vi "MB Registers Manager Write.vi"(5 "Data Reference":T2, 6 "Bits In":bool[](array[boolean]), 8 "error in (no error)":errorcluster, 9 "Words In":u16[](array[numeric]), 10 "Table":T1(ring), 11 "Start Address":u16) -> (0 "error out":errorcluster)   [LabVIEW 2019, in "NI_modbus_upd.lvlib"]
uses:
  NI_modbus_upd.lvlib
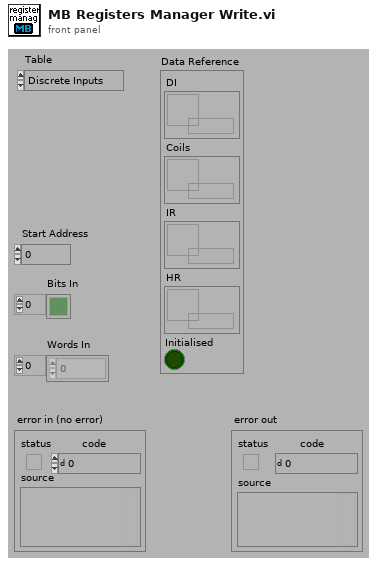
[diagram p1: front panel]
types:
  T1 = enum16{"Discrete Inputs", "Coils", "Input Registers", "Holding Registers"}
  T2 = cluster{"DI":refnum<data-value>, "Coils":refnum<data-value>, "IR":refnum<data-value>, "HR":refnum<data-value>, "Initialised":bool}
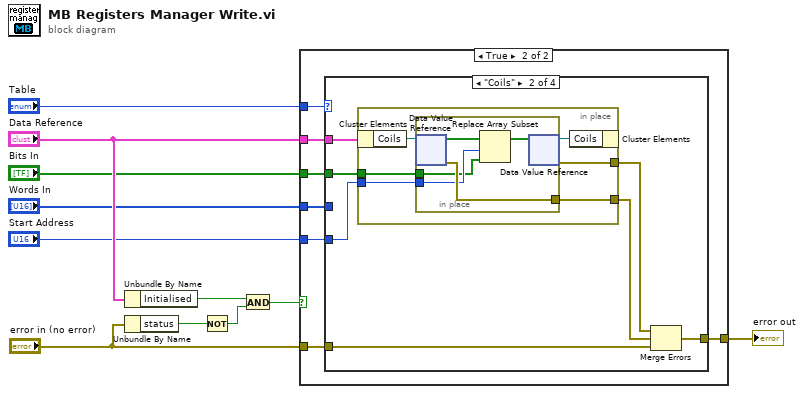
[diagram p0: block diagram]
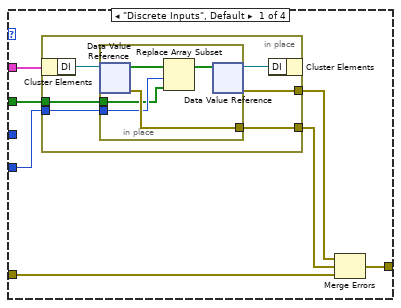
[diagram p3: hidden frame]
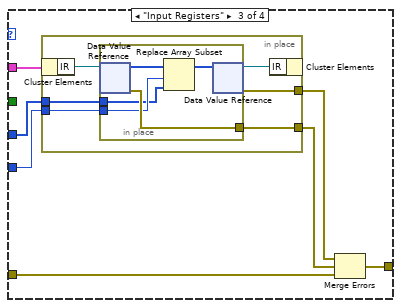
[diagram p4: hidden frame]
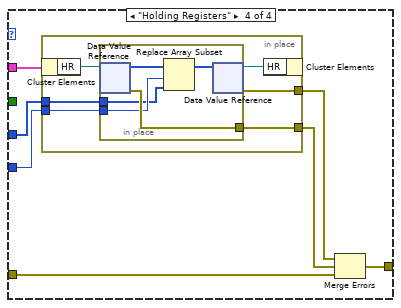
[diagram p5: hidden frame]
diagram:
  n1 = Unbundle By Name("Data Reference") -> ("Initialised"=w9:bool)
  n2 = Unbundle By Name("error in (no error)") -> ("status"=w11:bool)
  n3 = Not(x=w11) -> (.not. x?=w10:bool)
  n4 = And(x=w9, y=w10) -> (x .and. y?=w4:bool)
  n5 = case shown="True" w4 {
    tunnel: [w12 w16] -> w5
    tunnel: "Start Address" -> [_ w19]
    tunnel: "Table" -> [_ w15]
    tunnel: "Data Reference" -> [_ w18]
    tunnel: "error in (no error)" -> [w12 w17]
    tunnel: "Bits In" -> [_ w14]
    tunnel: "Words In" -> [_ w13]
    frame False {
    }
    frame True {
      n6 = case shown="\"Coils\"" w15 {
        tunnel: w19 -> [w26 w44 w62 w80]
        tunnel: w18 -> [w21 w39 w57 w75]
        tunnel: w17 -> [w25 w43 w61 w79]
        tunnel: [w22 w40 w58 w76] -> w16
        tunnel: w14 -> [w20 w38 _ _]
        tunnel: w13 -> [_ _ w56 w74]
        frame "Discrete Inputs", Default {
          n7 = in-place {
            in-place-border: w26 -> [w32]
            in-place-border: [w31] -> w24
            in-place-border: [w30] -> w23
            in-place-border: w20 -> [w27]
            n8 = in-place-cluster #1(w21) -> ("DI"=w29:refnum<data-value>)
            n9 = in-place {
              in-place-border: w32 -> [w34]
              in-place-border: [w37] -> w30
              in-place-border: w27 -> [w33]
              n10 = in-place-dvr #2(w29) -> (w36:bool[], w37:errorcluster)
              n11 = Replace Array Subset(array=w36, new element=w33, index=w34) -> (w35:bool[])
              n12 = in-place-dvr #2(w35) -> (w28:refnum<data-value>, w31:errorcluster)
            }
            n13 = in-place-cluster #1("DI"=w28) -> ()  [unwired: 1 out]
          }
          n14 = Merge Errors(w24, w23, w25) -> (w22:errorcluster)
        }
        frame "Coils" {
          n15 = in-place {
            in-place-border: w44 -> [w50]
            in-place-border: [w49] -> w42
            in-place-border: [w48] -> w41
            in-place-border: w38 -> [w45]
            n16 = in-place-cluster #3(w39) -> ("Coils"=w47:refnum<data-value>)
            n17 = in-place {
              in-place-border: w50 -> [w52]
              in-place-border: [w55] -> w48
              in-place-border: w45 -> [w51]
              n18 = in-place-dvr #4(w47) -> (w54:bool[], w55:errorcluster)
              n19 = Replace Array Subset(array=w54, new element=w51, index=w52) -> (w53:bool[])
              n20 = in-place-dvr #4(w53) -> (w46:refnum<data-value>, w49:errorcluster)
            }
            n21 = in-place-cluster #3("Coils"=w46) -> ()  [unwired: 1 out]
          }
          n22 = Merge Errors(w42, w41, w43) -> (w40:errorcluster)
        }
        frame "Input Registers" {
          n23 = in-place {
            in-place-border: w62 -> [w68]
            in-place-border: [w67] -> w60
            in-place-border: [w66] -> w59
            in-place-border: w56 -> [w63]
            n24 = in-place-cluster #5(w57) -> ("IR"=w65:refnum<data-value>)
            n25 = in-place {
              in-place-border: w68 -> [w70]
              in-place-border: [w73] -> w66
              in-place-border: w63 -> [w69]
              n26 = in-place-dvr #6(w65) -> (w72:u16[], w73:errorcluster)
              n27 = Replace Array Subset(array=w72, new element=w69, index=w70) -> (w71:u16[])
              n28 = in-place-dvr #6(w71) -> (w64:refnum<data-value>, w67:errorcluster)
            }
            n29 = in-place-cluster #5("IR"=w64) -> ()  [unwired: 1 out]
          }
          n30 = Merge Errors(w60, w59, w61) -> (w58:errorcluster)
        }
        frame "Holding Registers" {
          n31 = in-place {
            in-place-border: w80 -> [w86]
            in-place-border: [w85] -> w78
            in-place-border: [w84] -> w77
            in-place-border: w74 -> [w81]
            n32 = in-place-cluster #7(w75) -> ("HR"=w83:refnum<data-value>)
            n33 = in-place {
              in-place-border: w86 -> [w88]
              in-place-border: [w91] -> w84
              in-place-border: w81 -> [w87]
              n34 = in-place-dvr #8(w83) -> (w90:u16[], w91:errorcluster)
              n35 = Replace Array Subset(array=w90, new element=w87, index=w88) -> (w89:u16[])
              n36 = in-place-dvr #8(w89) -> (w82:refnum<data-value>, w85:errorcluster)
            }
            n37 = in-place-cluster #7("HR"=w82) -> ()  [unwired: 1 out]
          }
          n38 = Merge Errors(w78, w77, w79) -> (w76:errorcluster)
        }
      }
    }
  }
  "error out" <- w5
